vi "Chain of Responsibility Example.vi"() -> ()   [LabVIEW 2017, in "Chain of Responsiblility Example.lvlib"]
doc: "### Chain of Responsibility Example(Chain of Responsibility Example.vi)\n\n#### Overview\n\nDemonstrates the responsibility chain design pattern implemented in the CSM framework. By clicking the buttons on the front panel, you can observe how the responsibility chain processes allowed messages in a defined sequence.\n\nEach message is passed through the chain from the lowest-ordered module to the highest-ordered module. Processing stops when a module successfully handles the message, and the message is not forwarded to subsequent modules. If no module in the chain can process the message, this example returns an error.\n\n#### Introduction\n\nThis example demonstrates the responsibility chain mode in the CSM framework. Responsibility chain CSM module should always be marked with a \"$\" and an integer number as suffix, such as \"CSMName$1\", \"CSMName$2\", and so on. \n\nA group of responsibility chain CSM modules process messages both in allowed ways and also in a sequential order:\n\n- Only specially allowed messages can be processed by each individual chain module.\n- If one message is allowed by multiple chain modules, the chain module with the lowest order will process the message and the message won't be processed by higher-ordered chain module any more.\n\n#### Instructions\n\n1. Run this VI.\n2. Click any of the buttons on the front panel, such as \"Action: action 1 -> Chain\", then you can see which chain module has processed which message. \n3. Click the \"Macro: Exit -> Chain\" or \"Macro: Exit -@ Chain\" button, then you can see the chain module will be initiated in an ordered way.\n\n#### Steps\n\nStep 1: Add special allowed messages for each individual CSM submodule which will be then marked with chain mode, such as \"Action: action 1\" and \"Action: action 2\" for the \"Chain$1\" CSM submodule in this example.\n\nStep 2: Drop a template CSM VI with UI and name it as ChainModeExample. \n\nStep 3: Create boolean buttons in the UI, such as \"Action: action 1 -> Chain\" and so on to simulate the inter-module message transfer. \n\nStep 4: Use high-level APIs to monitor the status of all running CSM modules.\n\nStep 5: Use global log APIs to calculate and monitor the real-time logging capability, please refer to 4. Advance Examples\\6. Global Log Handling Capability for more details."
uses:
  Chain of Responsiblility Example.lvlib
  user.lib/_NEVSTOP/Communicable State Machine(CSM)/Utility/_support/Periodic String Filter Level.ctl
  user.lib/_NEVSTOP/Communicable State Machine(CSM)/_Support/Typedef/_CSM_MODE.ctl
  user.lib/_NEVSTOP/Communicable State Machine(CSM)/Utility/Periodic String Filter Setting.ctl
  user.lib/_NEVSTOP/Communicable State Machine(CSM)/AdvanceAPI/CSM - Revert Arguments-Safe String.vi
  user.lib/_NEVSTOP/Communicable State Machine(CSM)/AdvanceAPI/CSM - Make String Arguments Safe.vi
  user.lib/_NEVSTOP/Communicable State Machine(CSM)/AdvanceAPI/CSM - Break Down Multiple States String.vi
  user.lib/_NEVSTOP/Communicable State Machine(CSM)/AdvanceAPI/CSM - Compact Multiple States.vi
  user.lib/_NEVSTOP/Communicable State Machine(CSM)/AdvanceAPI/CSM - Keywords.vi
  user.lib/_NEVSTOP/Communicable State Machine(CSM)/_Shared/Trim Single-line Text.vi
  user.lib/_NEVSTOP/Communicable State Machine(CSM)/Communicable State Machine.lvlib
  user.lib/_NEVSTOP/Communicable State Machine(CSM)/_Shared/CSM Shared.lvlib
panel:
  out "Array":T2(array[cluster])
  in  "All?":bool
  out "LogInQ":i32
  out "State History 2":string
  out "log handling Speed(#/s)":dbl
  out "LogInQ changing Speed(#/s)":dbl
  out "Level":T3
  in  "Macro: Exit -@ Chain":bool
  in  "Macro: Exit -> Chain":bool
  in  "Action: action 6 -@ Chain":bool
  in  "Action: action 5 -@ Chain":bool
  in  "Action: action 4 -@ Chain":bool
  in  "Action: action 3 -@ Chain":bool
  in  "Action: action 2 -@ Chain":bool
  in  "Action: action 1 -@ Chain":bool
  in  "Action: action 6 -> Chain":bool
  in  "Action: action 5 -> Chain":bool
  in  "Action: action 4 -> Chain":bool
  in  "Action: action 3 -> Chain":bool
  in  "Action: action 2 -> Chain":bool
  in  "Action: action 1 -> Chain":bool
  out "State History":string
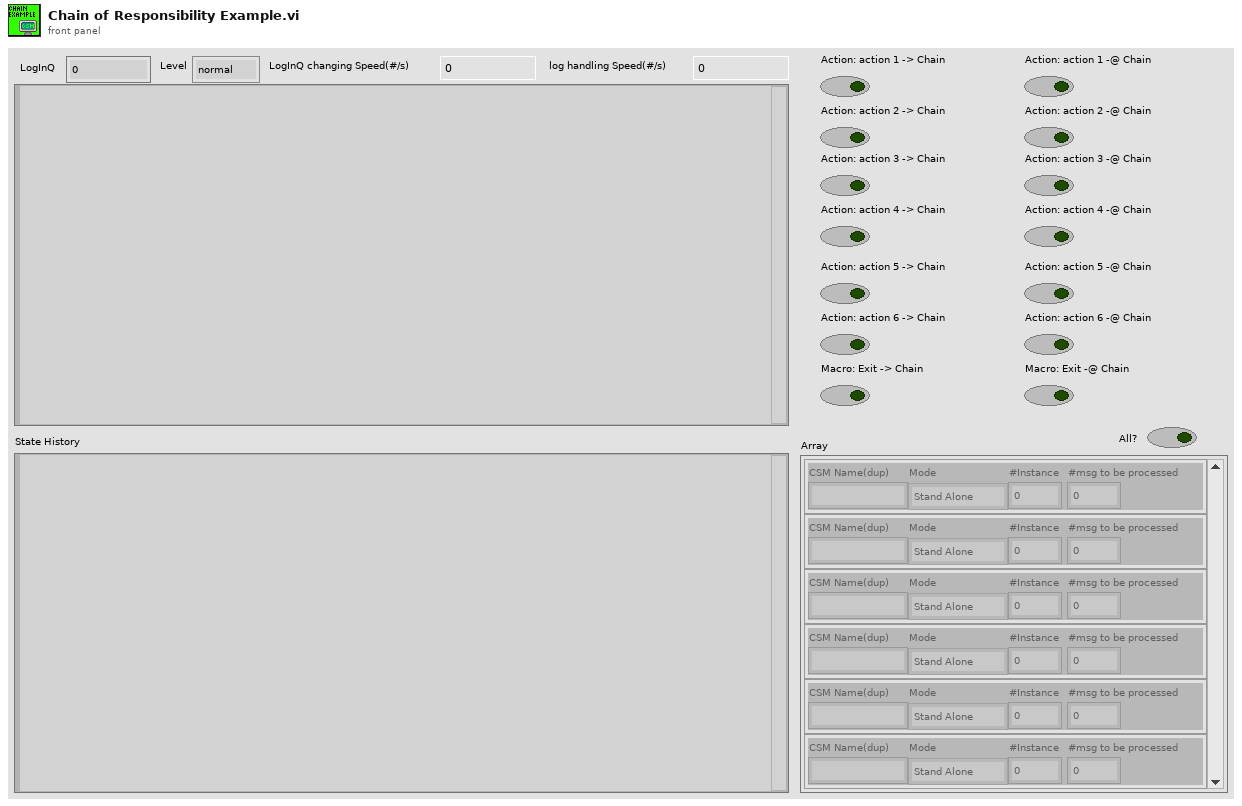
[diagram p1: front panel]
types:
  T1 = typedef "Communicable State Machine.lvlib/_CSM_MODE.ctl" = enum16{"Not Exist", "Stand Alone", "CSM", "Worker", "Worker Agent", "Chain Node", "Chain"}
  T2 = cluster{"CSM Name(dup)":string, "Mode":T1, "#Instance":i32, "#msg to be processed":i32}[]
  T3 = typedef "Communicable State Machine.lvlib/Periodic String Filter Level.ctl" = enum16{"normal", "L1", "L2", "L3", "L4"}
  T4 = enum32{"Invalid", "Standard", "Closed", "Hidden", "Minimized", "Maximized"}
  T5 = enum32{"invalid app kind", "Development System", "Run Time System", "Student Edition", "Embedded LabVIEW", "Evaluation", "Custom"}
  T6 = typedef "Communicable State Machine.lvlib/_CSM_Response Source Message.ctl" = cluster{"‘State":string, "’Arguments":string, "’Error":errorcluster}
  T7 = cluster{"Current VI Reference":refnum<vi>, "Close Panel on Exit?":bool}
  T8 = cluster{"Core":cluster{"Current VI Reference":refnum<vi>, "Close Panel on Exit?":bool}, "Your Boolean data":bool, "Your string data":string}
  T9 = cluster{"CSM Name (Dup)":string, "Mode":T1, "#Instance":i32, "#Elements In Queue":i32}
  T10 = typedef "Communicable State Machine.lvlib/Periodic String Filter Setting.ctl" = cluster{"threashold(#/s)":dbl, "Check Peroid(s)":dbl}
  T11 = typedef "Communicable State Machine.lvlib/_CSM_GlobalLog_MSG.ctl" = cluster{"Name (\"\" to Use UUID)":string, "Current State":string, "Arguments":string, "Source Message":T6, "Source Module":string, "Complete(T)/Start(F)":bool, "LogType":T12, "Time Stamp":timestamp}
  T12 = typedef "Communicable State Machine.lvlib/_CSM_GlobalLog_MSG_TYPE.ctl" = enum16{"User Log", "State Change", "Status", "Interrupt", "Register", "Unregister", "Error Log", "Module Created", "Module Destroyed"}
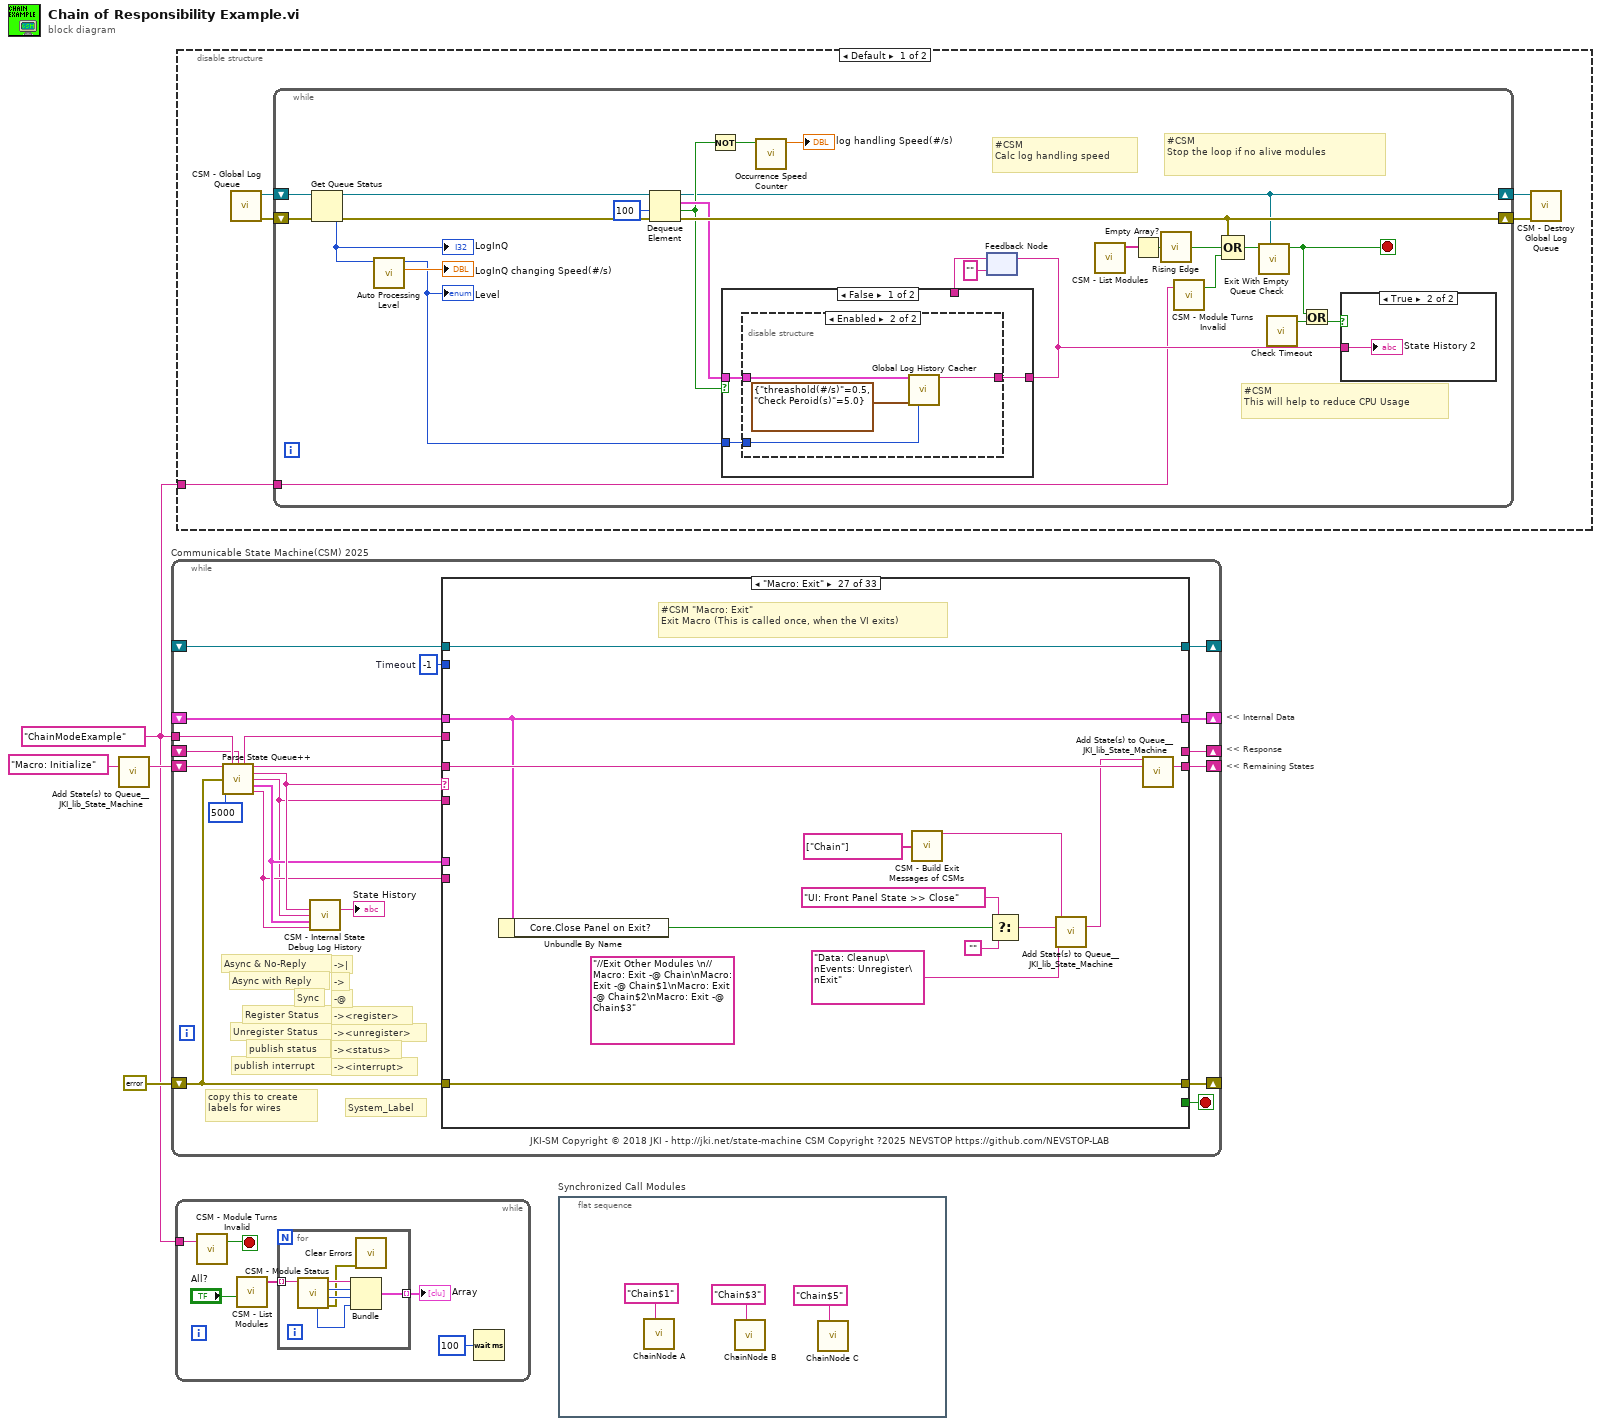
[diagram p0: block diagram]
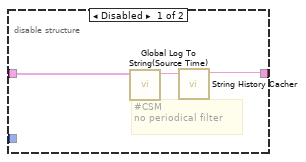
[diagram p2: hidden frame]
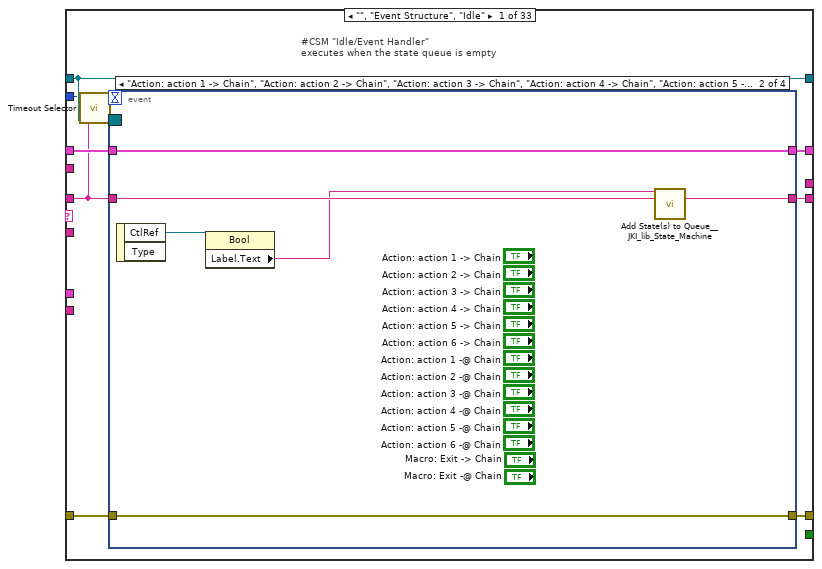
[diagram p6: hidden frame]
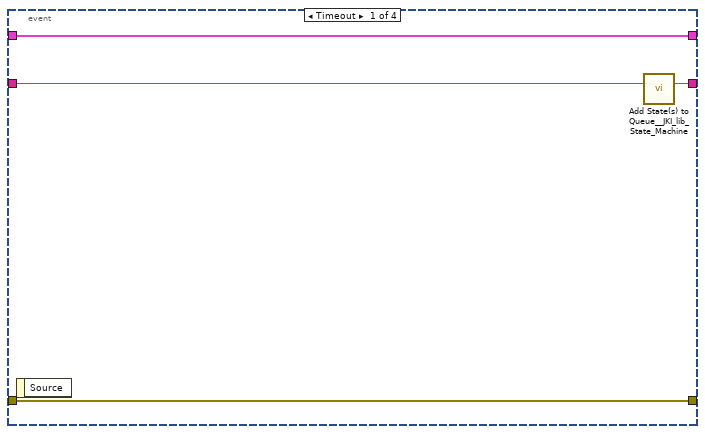
[diagram p7: hidden frame]
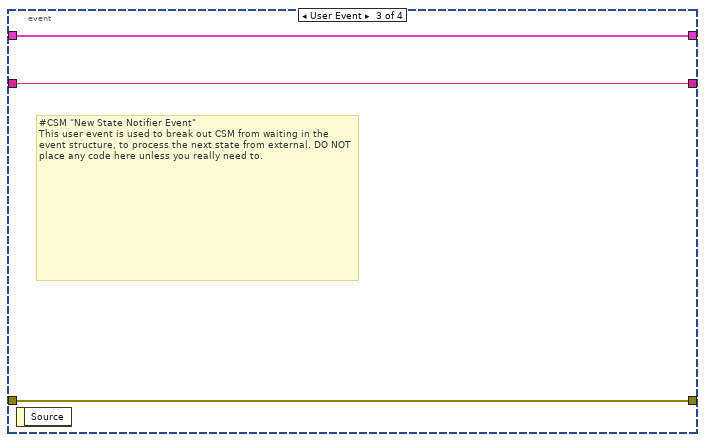
[diagram p8: hidden frame]
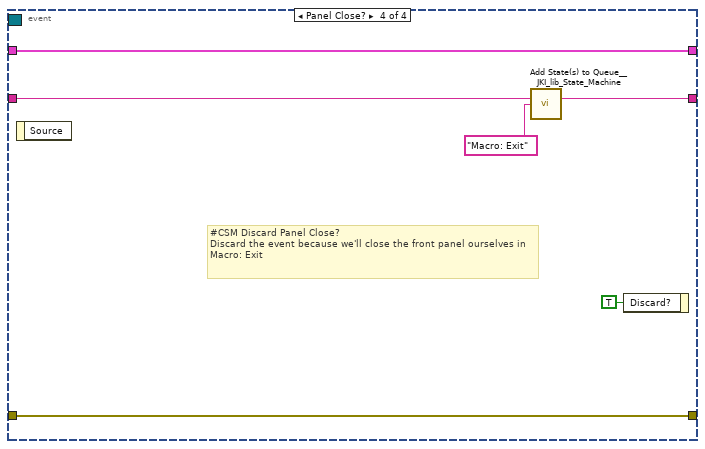
[diagram p9: hidden frame]
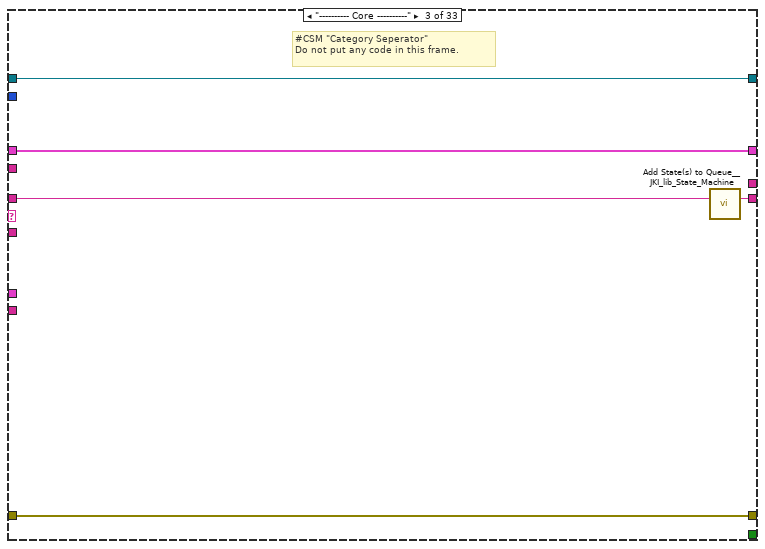
[diagram p11: hidden frame]
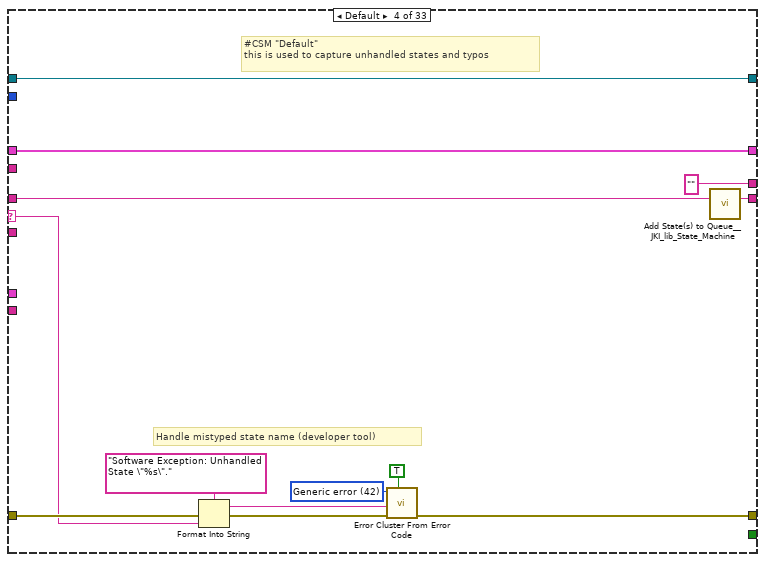
[diagram p12: hidden frame]
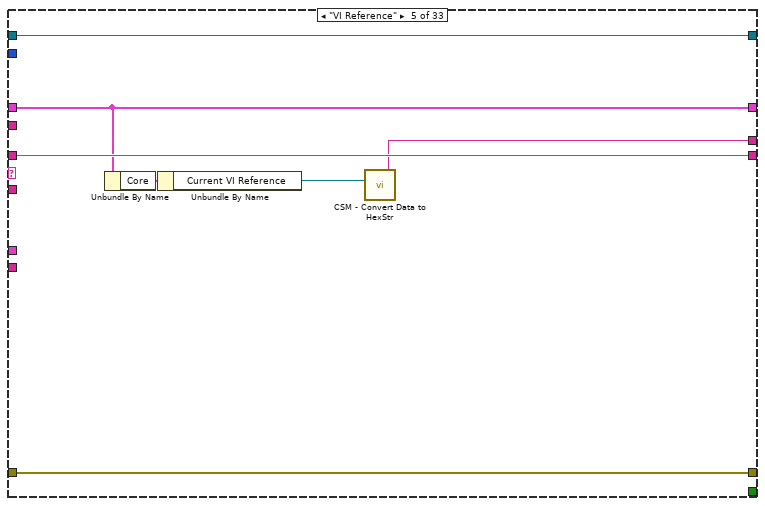
[diagram p13: hidden frame]
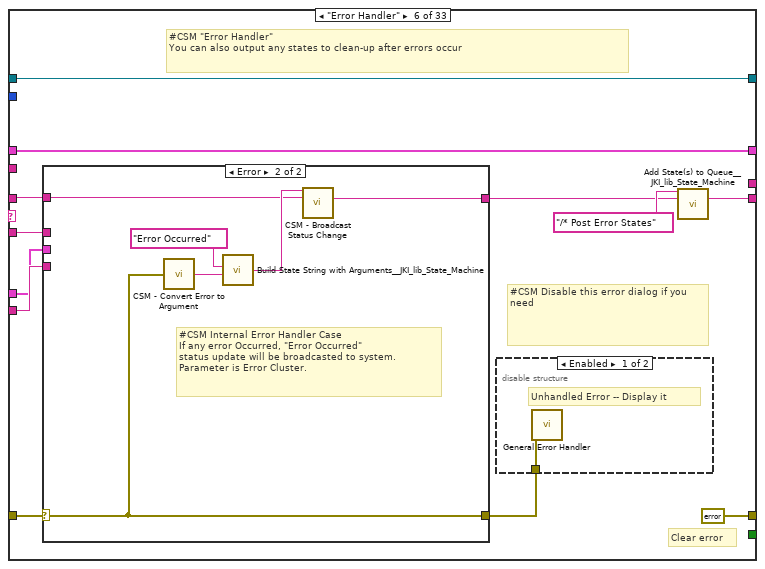
[diagram p14: hidden frame]
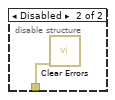
[diagram p15: hidden frame]
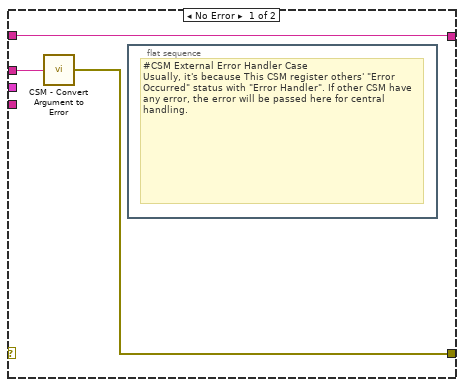
[diagram p16: hidden frame]
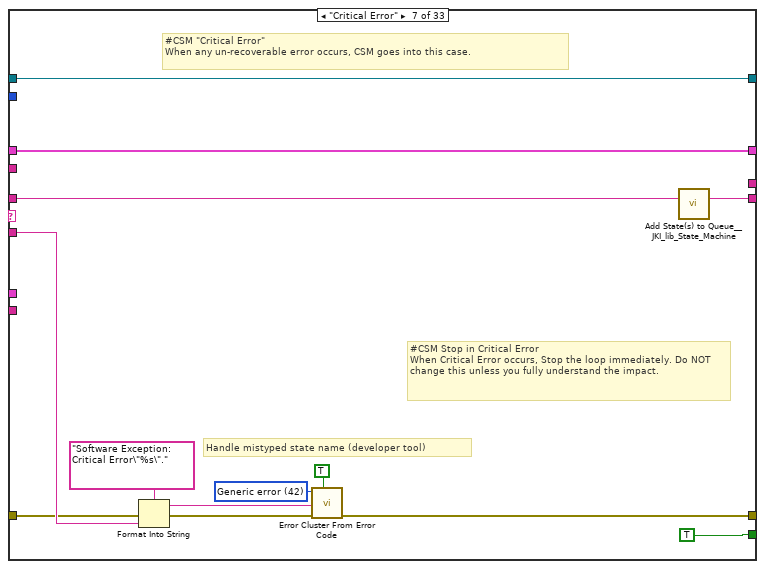
[diagram p17: hidden frame]
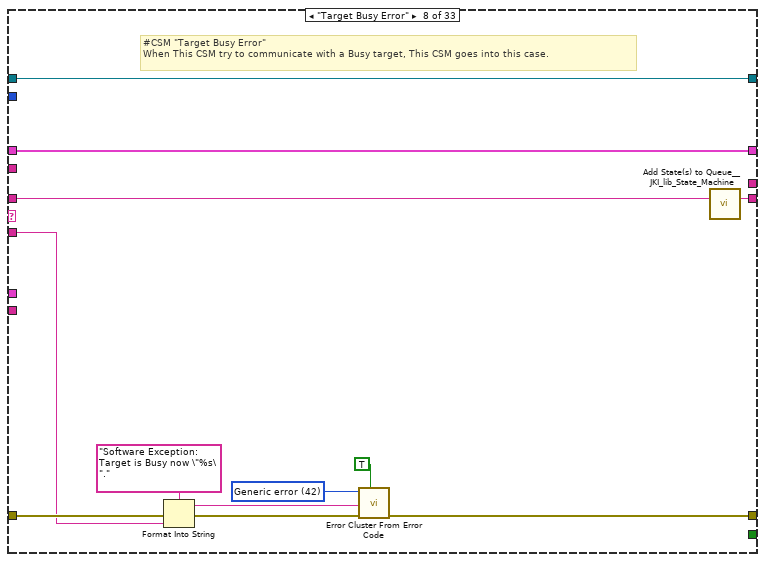
[diagram p18: hidden frame]
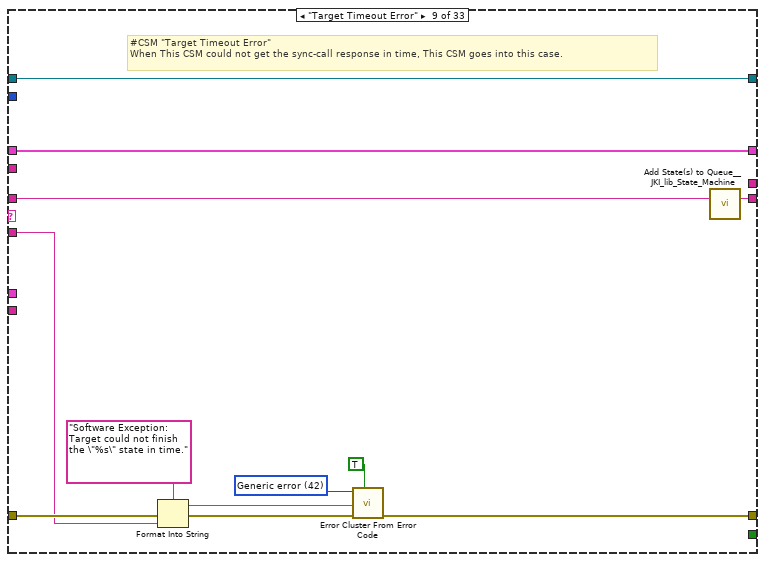
[diagram p19: hidden frame]
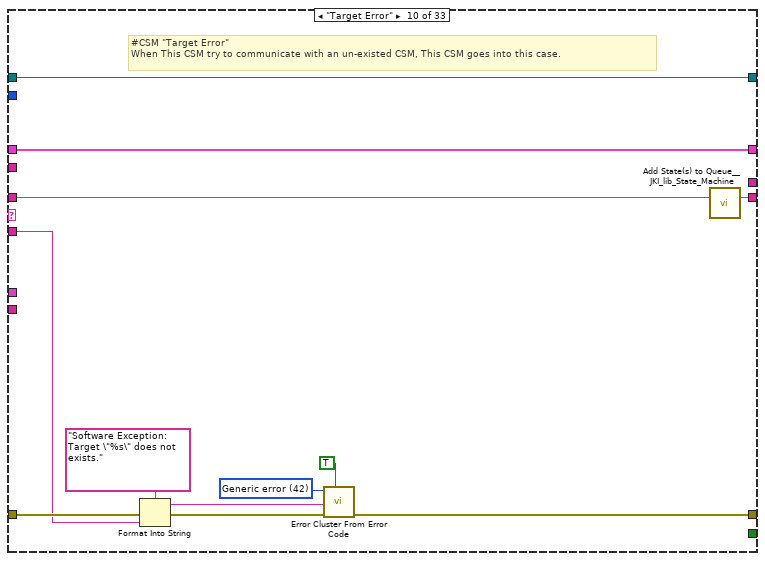
[diagram p20: hidden frame]
diagram:
  w1 = "ChainModeExample" ("Name (\"\" to Use UUID)")
  # "<< Internal Data"
  # "<< Response"
  # "<< Remaining States"
  n1 = call <vilib>:"Add State(s) to Queue__JKI_lib_State_Machine.vi"("State(s) in (\"\")"="Macro: Initialize" ("Init State(\"Macro: Initialize\")")) -> ("States Out"=w4:string)  [unwired: 14 in]
  n2 = while "Communicable State Machine(CSM) 2025" {
    shift-right: [w20] -> _
    shift-left: _ -> [w19]
    shift-right: [w23] -> _
    shift-left: errorcluster {"status"=FALSE, "code"=0, "source"=""} ("error out") -> [w17]
    shift-right: [w22] -> _
    shift-left: w4 -> [w24]
    tunnel: w1 -> [w12]
    shift-right: [w15] -> _
    shift-left: _ -> [w7]
    shift-right: [w14] -> _
    shift-left: _ -> [w13]
    stop <- w21 stop-if-true
    w18 = -1  # Timeout
    # "-><interrupt>"
    # "-><status>"
    # "-><unregister>"
    # "-><register>"
    # "-@"
    # "->"
    # "->|"
    # "publish interrupt"
    # "publish status"
    # "Unregister Status"
    # "Register Status"
    # "Sync"
    # "Async with Reply"
    # "Async & No-Reply"
    # "copy this to create labels for wires"
    # "System_Label"
    # "JKI-SM Copyright © 2018 JKI - http://jki.net/state-machine CSM Copyright ?2025 NEVSTOP https://github.com/NEVSTOP-LAB"
    n3 = call "Parse State Queue++.vi"("State Queue"=w24, "Name (\"\" to Use UUID)"=w12, "Response Arguments"=w7, "Previous Error"=w17, "Response Timeout (-2 Use Global Settings)"=5000 ("Response Timeout(1000ms)")) -> ("Name Used"=w8:string, "Remaining States"=w25:string, "Current State"=w11:string, "Arguments"=w6:string, ">> Response Source Message >>"=w10:T6, ">> Source CSM >>"=w9:string)  [unwired: 5 in]
    n4 = call "CSM - Internal State Debug Log History.vi"("State"=w11, "Arguments (\"\")"=w6, ">> Response Source Message >>"=w10, "Source (\"\")"=w9) -> ("Debug Log"=→"State History":string)  [unwired: 11 in]
    n5 = case shown="\"Macro: Exit\"" w11 {
      selector: w11 -> [_ _ _ w65 _ _ _ _ _ _ _ _ _ _ _ _ _ _ _ _ _ _ _ _ _ _ _ _ _ _ _ _ _]
      tunnel: w25 -> [w26 w57 w62 w69 w81 w87 w117 w120 w137 w149 w164 w173 w188 w194 w199 w207 w214 w219 w226 w230 w236 w241 w248 w264 w334 w340 w353 w356 w361 w365 w371 w376 w381]
      tunnel: w6 -> [_ _ _ _ _ w85 w110 w122 w133 w145 w158 _ _ _ _ _ _ _ _ _ _ _ w243 w258 _ _ _ _ _ _ _ _ _]
      tunnel: w19 -> [w33 w56 w59 w67 w80 w93 w118 w124 w135 w147 w162 w172 w181 w192 w196 _ w209 w216 w225 w229 w233 w239 w246 w260 w331 w337 w350 w355 w360 w364 w368 w373 w378]
      tunnel: [w32 w55 w60 w71 w82 errorcluster {"status"=FALSE, "code"=0, "source"=""} ("error out") w106 w119 w131 w143 w161 w174 w185 w191 w197 w204 w210 w217 w220 w228 w234 w238 w244 w261 w332 w338 w351 w357 w362 w366 w369 w374 w379] -> w23
      tunnel: w17 -> [w31 w55 w60 w70 w82 w91 w107 w126 w138 w150 _ w174 w185 w191 w197 w204 w211 w217 _ w231 w234 w238 w245 w262 w332 w338 w351 w357 w362 w366 w369 w374 w379]
      tunnel: [w34 w57 w61 w68 w81 w89 w116 w125 w136 w148 w165 w173 w187 w193 w198 w206 w213 w218 w226 w230 w235 w240 w247 w263 w333 w339 w352 w356 w361 w365 w370 w375 w380] -> w22
      tunnel: [_ _ _ _ _ _ TRUE _ _ _ _ _ _ TRUE _ _ _ _ _ _ _ _ _ _ _ _ _ _ _ _ _ _ _] -> w21
      tunnel: [w30 w56 w59 w67 w80 w93 w118 w124 w135 w147 w163 w172 w186 w192 w196 w205 w209 w216 w225 w229 w233 w239 w246 w260 w331 w337 w350 w355 w360 w364 w368 w373 w378] -> w20
      tunnel: w18 -> [w28 _ _ _ _ _ _ _ _ _ _ _ _ _ _ _ _ _ _ _ _ _ _ _ _ _ _ _ _ _ _ _ _]
      tunnel: w9 -> [_ _ _ _ _ w84 _ _ _ _ w159 _ _ _ _ _ _ _ _ _ _ _ _ _ _ _ _ _ _ _ _ _ _]
      tunnel: w10 -> [_ _ _ _ _ w83 _ _ _ _ w160 _ _ _ _ _ _ _ _ _ _ _ _ _ _ _ _ _ _ _ _ _ _]
      tunnel: [_ _ _ "" w76 _ _ _ _ _ _ _ _ _ _ _ _ _ _ _ _ _ _ _ _ _ _ _ "API1 Response" _ _ _ _] -> w15
      tunnel: [w29 w54 w58 w63 w79 w92 w108 w121 w132 w144 w166 w171 w175 w189 w195 w200 w208 w215 w224 w227 w232 w237 w242 w257 w330 w335 w343 w354 w359 w363 w367 w372 w377] -> w14
      tunnel: w13 -> [w29 w54 w58 w63 w79 w92 w108 w121 w132 w144 w166 w171 w175 w189 w195 w200 w208 w215 _ w227 w232 w237 w242 w257 w330 w335 w343 w354 w359 w363 w367 w372 w377]
      tunnel: w8 -> [_ _ _ _ _ _ _ _ _ _ _ _ _ _ _ _ _ _ w223 _ _ _ _ _ _ _ _ _ _ _ _ _ _]
      frame "", "Event Structure", "Idle" {
        # "#CSM \"Idle/Event Handler\"\nexecutes when the state queue is empty"
        n6 = call "Timeout Selector.vi"("Remaining States"=w26, "Timeout Expected"=w28) -> ("Timeout"=w27:i32)  [unwired: 5 in]
        n7 = event shown="[1] \"Action: action 1 -> Chain\", \"Action: action 2 -> Chain\", \"Action: action 3 -> Chain\", \"Action: action 4 -> Chain\", \"Action: action 5 -> Chain\", \"Action: action 6 -> Chain\", \"Action: action 1 -@ Chain\", \"Action: action 2 -@ Chain\", \"Action: action 3 -@ Chain\", \"Action: action 4 -@ Chain\", \"Action: action 5 -@ Chain\", \"Action: action 6 -@ Chain\", \"Macro: Exit -> Chain\", \"Macro: Exit -@ Chain\": Value Change" {
          selector: w29 -> [_ _ _ _]
          dyn-events: _ -> [_ _ _ _]
          timeout: w27 -> [_ _ _ _]
          tunnel: w26 -> [w38 w42 w46 w53]
          tunnel: [w37 w41 w46 w52] -> w34
          tunnel: w33 -> [w35 w43 w47 w50]
          tunnel: [w36 w44 w45 w51] -> w32
          tunnel: w31 -> [w36 w44 w45 w51]
          tunnel: [w35 w43 w47 w50] -> w30
          event Timeout {
            n8 = event-data() -> ()  [unwired: 1 in, 1 out]
            n9 = call <vilib>:"Add State(s) to Queue__JKI_lib_State_Machine.vi"("State(s) in (\"\")"=w38) -> ("States Out"=w37:string)  [unwired: 14 in]
          }
          event "Action: action 1 -> Chain", "Action: action 2 -> Chain", "Action: action 3 -> Chain", "Action: action 4 -> Chain", "Action: action 5 -> Chain", "Action: action 6 -> Chain", "Action: action 1 -@ Chain", "Action: action 2 -@ Chain", "Action: action 3 -@ Chain", "Action: action 4 -@ Chain", "Action: action 5 -@ Chain", "Action: action 6 -@ Chain", "Macro: Exit -> Chain", "Macro: Exit -@ Chain": Value Change {
            n10 = event-data() -> ("CtlRef"=w40:refnum<vi>)  [unwired: 1 in, 1 out]
            n11 = property class="Bool"(reference=w40) -> ("Label.Text"=w39:string)  [unwired: 1 in, 2 out]
            n12 = call <vilib>:"Add State(s) to Queue__JKI_lib_State_Machine.vi"("State(s) in Front (\"\")"=w39, "State(s) in (\"\")"=w42) -> ("States Out"=w41:string)  [unwired: 13 in]
          }
          event User Event {
            # "#CSM \"New State Notifier Event\"\nThis user event is used to break out CSM from waiting in the event structure, to process the next state from external. DO NOT place any code here unless you really need to."
            n13 = event-data() -> ()  [unwired: 1 in, 1 out]
          }
          event Panel Close? {
            # "#CSM Discard Panel Close?\nDiscard the event because we'll close the front panel ourselves in Macro: Exit"
            n14 = event-data() -> ()  [unwired: 1 in, 1 out]
            n15 = call <vilib>:"Add State(s) to Queue__JKI_lib_State_Machine.vi"("State(s) in (\"\")"=w53, "State(s) at Back (\"\")"="Macro: Exit") -> ("States Out"=w52:string)  [unwired: 13 in]
            n16 = event-data("Discard?"=TRUE) -> ()  [unwired: 1 in, 1 out]
          }
        }
      }
      frame "CSM Documentation" {
        # "#CSM \"Documentation\"\nCase for holding CSM Documenation"
        # "CSM Documentation"
        # "#CSM Commenting\nTo add a comment use \"//\" or \"#\" and all text to the right will be ignored\n\nCommenting Example:\nUI: Initialize // This initializes the UI\n// Another comment line"
        # "#CSM State Syntax\n\n    // Local Message Example\n    DoSth: DoA >> Arguments\n\n    // Sync Call Example\n    API: xxxx >> Arguments -@ TargetModule\n\n    // Async Call Example\n    API: xxxx >> Arguments -> TargetModule\n\n    // Async Call without Reply Example\n    API: xxxx >> Arguments ->| TargetModule\n\n    // Broadcast normal status:\n    Status >> StatusArguments  -><status>\n\n    // Broadcast Interrupt status:\n    Interrupt >> StatusArguments  -><interrupt>\n\n    // Register Source Module's status to Handler Module\n    Status@Source Module >> Handler Module@Handler Module -><register>\n\n    // Unegister Source Module's status\n    Status@Source Module >> Handler Module -><unregister>"
        # "#CSM README FIRST\n\nCSM is a LabVIEW application framework that builds upon JKI State Machine (CSM). It follows the pattern of CSM and extends the keywords to describe message communication between CSM modules, including concepts such as Sync-Message, Async-Message, Subscription/Unsubscription of status - essential elements for creating reusable code modules. For more information, please visit the CSM wiki: https://github.com/NEVSTOP-LAB/JKI-State-Machine-Plus-Plus/wiki\n\nFor instructions on JKI State Machine, visit: \n    http://jki.net/state-machine/\nFor information about CSM, visit: \n    https://github.com/NEVSTOP-LAB"
      }
      frame "---------- Core ----------" {
        # "#CSM \"Category Seperator\"\nDo not put any code in this frame."
        n17 = call <vilib>:"Add State(s) to Queue__JKI_lib_State_Machine.vi"("State(s) in (\"\")"=w62) -> ("States Out"=w61:string)  [unwired: 14 in]
      }
      frame Default {
        w74 = 42 items=["No error", "Argument error", "Memory is full", "Out of zone", "End of file", "File already open", "Generic file I/O error", "File not found", "File permission error", "Disk is full", "Duplicate path", "Too many files open", "System feature not enabled", "Resource file not found", "Cannot add resource", "Resource not found", "Image not found", "Image memory error", "Pen does not exist", "Config type invalid", "Config token not found", "Config parse error", "Config memory error", "Bad external code format", "Bad external code offset", "External code not present", "Null window", "Destroy window error", "Null menu", "Print aborted", "Bad print record", "Print driver error", "Windows error during printing", "Memory error during printing", "Print dialog error", "Generic print error", "Invalid device refnum", "Device not found", "Device parameter error", "Device unit error", "Cannot open device", "Device call aborted", "Generic error", "Cancelled by user", "Object ID too low", "Object ID too high", "Object not in heap", "Unknown heap", "Unknown object (invalid DefProc)", "Unknown object (DefProc not in table)", "Message out of range", "Invalid (null) method", "Unknown message", "Manager call not supported", "Bad address", "Network operation in progress", "Network operation timed out", "Connection is busy", "Network attribute not supported", "Network error", "Address in use", "System out of memory", "Connection aborted", "Connection refused", "Not connected", "Already connected", "Connection closed", "Initialization error (interapplication manager)", "Bad occurrence", "Wait on unbound occurrence handler", "Occurrence queue overflow", "Datalog type conflict", "Unused", "Unrecognized type (interapplication manager)", "Memory corrupt", "Failed to make temporary DLL", "Old CIN version", "Drag socket not found", "Failed to load drop-object", "Failed to register OLE object", "Failed to release OLE object", "Format specifier type mismatch", "Unknown format specifier", "Too few format specifiers", "Too many format specifiers", "Scan failed", "Newer CIN version", "Error converting to variant", "Runtime menu error", "Password tampered", "Variant attribute not found", "Incompatible variant data type", "Event data is not available", "Event Store is not present", "Occurrence is not found", "Event Queue is not created", "Event info is not available", "Refnum passed is NULL", "Error retrieving Class GUID", "Error retrieving CoClass GUID", "Error retrieving TypeLib GUID.", "Bad built application magic bytes.", "Specific driver is different from the specific driver associated with the Logical Name.", "There is no session opened to the class driver.", "Max Error", "MAX - Error with config objects", "MAX - Error loading configuration", "MAX - Group not supported"]
        # "#CSM \"Default\"\nthis is used to capture unhandled states and typos"
        # "Handle mistyped state name (developer tool)"
        n18 = Format Into String(format string="Software Exception: Unhandled State \"%s\"." ("message"), error in=w70, w65) -> (resulting string=w73:string, error out=w72:errorcluster)  [unwired: 1 in]
        n19 = call <vilib>:"Error Cluster From Error Code.vi"("show call chain? (False)"=TRUE, "error in (no error)"=w72, "error message (\"\")"=w73, "error code (0)"=w74) -> ("error out"=w71:errorcluster)  [unwired: 5 in]
        n20 = call <vilib>:"Add State(s) to Queue__JKI_lib_State_Machine.vi"("State(s) in (\"\")"=w69) -> ("States Out"=w68:string)  [unwired: 14 in]
      }
      frame "VI Reference" {
        n21 = Unbundle By Name(w80) -> ("Core"=w78:T7)
        n22 = Unbundle By Name(w78) -> ("Current VI Reference"=w77:refnum<vi>)
        n23 = call "CSM - Convert Data to HexStr.vi"("Variant"=w77) -> ("HEX String (0-9,A-F)"=w76:string)  [unwired: 8 in]
      }
      frame "Error Handler" {
        # "#CSM Disable this error dialog if you need"
        # "#CSM \"Error Handler\"\nYou can also output any states to clean-up after errors occur"
        # "Clear error"
        n24 = case shown="Error" w91 {
          selector: w91 -> [_ w100]
          tunnel: [w98 w102] -> w88
          tunnel: w87 -> [w98 w101]
          tunnel: [w97 w100] -> w86
          tunnel: w85 -> [w99 _]
          tunnel: w84 -> [_ _]
          tunnel: w83 -> [_ _]
          frame No Error {
            n25 = call "CSM - Convert Argument to Error.vi"("Argument"=w99) -> ("Error"=w97:errorcluster)  [unwired: 4 in]
            n26 = flat-sequence {
              frame #0 {
                # "#CSM External Error Handler Case\nUsually, it's because This CSM register others' \"Error Occurred\" status with \"Error Handler\". If other CSM have any error, the error will be passed here for central handling."
              }
            }
          }
          frame Error {
            # "#CSM Internal Error Handler Case \nIf any error Occurred, \"Error Occurred\" \nstatus update will be broadcasted to system.\nParameter is Error Cluster."
            n27 = call "CSM - Convert Error to Argument.vi"("Error"=w100) -> ("Argument"=w104:string)  [unwired: 4 in]
            n28 = call <vilib>:"Build State String with Arguments__JKI_lib_State_Machine.vi"("Arguments (\"\")"=w104, "State"="Error Occurred" ("Status with Arguments")) -> ("State with Arguments"=w103:string)  [unwired: 4 in]
            n29 = call "CSM - Broadcast Status Change.vi"("Status With Arguments"=w103, "State Queue"=w101) -> ("Remaining States"=w102:string)  [unwired: 13 in]
          }
        }
        n30 = disable-structure shown="Enabled" {
          disable-tunnel: w86 -> [w95 w96]
          frame Enabled {
            # "Unhandled Error -- Display it"
            n31 = call <vilib>:"General Error Handler.vi"("error in (no error)"=w95) -> ()  [unwired: 10 in, 5 out]
          }
          frame Disabled {
            n32 = call <vilib>:"Clear Errors.vi"("error in (no error)"=w96) -> ()  [unwired: 5 in, 2 out]
          }
        }
        n33 = call <vilib>:"Add State(s) to Queue__JKI_lib_State_Machine.vi"("State(s) in Front (\"\")"="/* Post Error States", "State(s) in (\"\")"=w88) -> ("States Out"=w89:string)  [unwired: 13 in]
      }
      frame "Critical Error" {
        w114 = 42 items=["No error", "Argument error", "Memory is full", "Out of zone", "End of file", "File already open", "Generic file I/O error", "File not found", "File permission error", "Disk is full", "Duplicate path", "Too many files open", "System feature not enabled", "Resource file not found", "Cannot add resource", "Resource not found", "Image not found", "Image memory error", "Pen does not exist", "Config type invalid", "Config token not found", "Config parse error", "Config memory error", "Bad external code format", "Bad external code offset", "External code not present", "Null window", "Destroy window error", "Null menu", "Print aborted", "Bad print record", "Print driver error", "Windows error during printing", "Memory error during printing", "Print dialog error", "Generic print error", "Invalid device refnum", "Device not found", "Device parameter error", "Device unit error", "Cannot open device", "Device call aborted", "Generic error", "Cancelled by user", "Object ID too low", "Object ID too high", "Object not in heap", "Unknown heap", "Unknown object (invalid DefProc)", "Unknown object (DefProc not in table)", "Message out of range", "Invalid (null) method", "Unknown message", "Manager call not supported", "Bad address", "Network operation in progress", "Network operation timed out", "Connection is busy", "Network attribute not supported", "Network error", "Address in use", "System out of memory", "Connection aborted", "Connection refused", "Not connected", "Already connected", "Connection closed", "Initialization error (interapplication manager)", "Bad occurrence", "Wait on unbound occurrence handler", "Occurrence queue overflow", "Datalog type conflict", "Unused", "Unrecognized type (interapplication manager)", "Memory corrupt", "Failed to make temporary DLL", "Old CIN version", "Drag socket not found", "Failed to load drop-object", "Failed to register OLE object", "Failed to release OLE object", "Format specifier type mismatch", "Unknown format specifier", "Too few format specifiers", "Too many format specifiers", "Scan failed", "Newer CIN version", "Error converting to variant", "Runtime menu error", "Password tampered", "Variant attribute not found", "Incompatible variant data type", "Event data is not available", "Event Store is not present", "Occurrence is not found", "Event Queue is not created", "Event info is not available", "Refnum passed is NULL", "Error retrieving Class GUID", "Error retrieving CoClass GUID", "Error retrieving TypeLib GUID.", "Bad built application magic bytes.", "Specific driver is different from the specific driver associated with the Logical Name.", "There is no session opened to the class driver.", "Max Error", "MAX - Error with config objects", "MAX - Error loading configuration", "MAX - Group not supported"]
        # "#CSM \"Critical Error\"\nWhen any un-recoverable error occurs, CSM goes into this case."
        # "#CSM Stop in Critical Error\nWhen Critical Error occurs, Stop the loop immediately. Do NOT change this unless you fully understand the impact."
        # "Handle mistyped state name (developer tool)"
        n34 = Format Into String(format string="Software Exception: Critical Error\"%s\"." ("message"), error in=w107, w110) -> (resulting string=w113:string, error out=w112:errorcluster)  [unwired: 1 in]
        n35 = call <vilib>:"Error Cluster From Error Code.vi"("show call chain? (False)"=TRUE, "error in (no error)"=w112, "error message (\"\")"=w113, "error code (0)"=w114) -> ("error out"=w106:errorcluster)  [unwired: 5 in]
        n36 = call <vilib>:"Add State(s) to Queue__JKI_lib_State_Machine.vi"("State(s) in (\"\")"=w117) -> ("States Out"=w116:string)  [unwired: 14 in]
      }
      frame "Target Busy Error" {
        w129 = 42 items=["No error", "Argument error", "Memory is full", "Out of zone", "End of file", "File already open", "Generic file I/O error", "File not found", "File permission error", "Disk is full", "Duplicate path", "Too many files open", "System feature not enabled", "Resource file not found", "Cannot add resource", "Resource not found", "Image not found", "Image memory error", "Pen does not exist", "Config type invalid", "Config token not found", "Config parse error", "Config memory error", "Bad external code format", "Bad external code offset", "External code not present", "Null window", "Destroy window error", "Null menu", "Print aborted", "Bad print record", "Print driver error", "Windows error during printing", "Memory error during printing", "Print dialog error", "Generic print error", "Invalid device refnum", "Device not found", "Device parameter error", "Device unit error", "Cannot open device", "Device call aborted", "Generic error", "Cancelled by user", "Object ID too low", "Object ID too high", "Object not in heap", "Unknown heap", "Unknown object (invalid DefProc)", "Unknown object (DefProc not in table)", "Message out of range", "Invalid (null) method", "Unknown message", "Manager call not supported", "Bad address", "Network operation in progress", "Network operation timed out", "Connection is busy", "Network attribute not supported", "Network error", "Address in use", "System out of memory", "Connection aborted", "Connection refused", "Not connected", "Already connected", "Connection closed", "Initialization error (interapplication manager)", "Bad occurrence", "Wait on unbound occurrence handler", "Occurrence queue overflow", "Datalog type conflict", "Unused", "Unrecognized type (interapplication manager)", "Memory corrupt", "Failed to make temporary DLL", "Old CIN version", "Drag socket not found", "Failed to load drop-object", "Failed to register OLE object", "Failed to release OLE object", "Format specifier type mismatch", "Unknown format specifier", "Too few format specifiers", "Too many format specifiers", "Scan failed", "Newer CIN version", "Error converting to variant", "Runtime menu error", "Password tampered", "Variant attribute not found", "Incompatible variant data type", "Event data is not available", "Event Store is not present", "Occurrence is not found", "Event Queue is not created", "Event info is not available", "Refnum passed is NULL", "Error retrieving Class GUID", "Error retrieving CoClass GUID", "Error retrieving TypeLib GUID.", "Bad built application magic bytes.", "Specific driver is different from the specific driver associated with the Logical Name.", "There is no session opened to the class driver.", "Max Error", "MAX - Error with config objects", "MAX - Error loading configuration", "MAX - Group not supported"]
        # "#CSM \"Target Busy Error\"\nWhen This CSM try to communicate with a Busy target, This CSM goes into this case."
        n37 = Format Into String(format string="Software Exception: Target is Busy now \"%s\"." ("message"), error in=w126, w122) -> (resulting string=w128:string, error out=w127:errorcluster)  [unwired: 1 in]
        n38 = call <vilib>:"Error Cluster From Error Code.vi"("show call chain? (False)"=TRUE, "error in (no error)"=w127, "error message (\"\")"=w128, "error code (0)"=w129) -> ("error out"=w119:errorcluster)  [unwired: 5 in]
        n39 = call <vilib>:"Add State(s) to Queue__JKI_lib_State_Machine.vi"("State(s) in (\"\")"=w120) -> ("States Out"=w125:string)  [unwired: 14 in]
      }
      frame "Target Timeout Error" {
        w141 = 42 items=["No error", "Argument error", "Memory is full", "Out of zone", "End of file", "File already open", "Generic file I/O error", "File not found", "File permission error", "Disk is full", "Duplicate path", "Too many files open", "System feature not enabled", "Resource file not found", "Cannot add resource", "Resource not found", "Image not found", "Image memory error", "Pen does not exist", "Config type invalid", "Config token not found", "Config parse error", "Config memory error", "Bad external code format", "Bad external code offset", "External code not present", "Null window", "Destroy window error", "Null menu", "Print aborted", "Bad print record", "Print driver error", "Windows error during printing", "Memory error during printing", "Print dialog error", "Generic print error", "Invalid device refnum", "Device not found", "Device parameter error", "Device unit error", "Cannot open device", "Device call aborted", "Generic error", "Cancelled by user", "Object ID too low", "Object ID too high", "Object not in heap", "Unknown heap", "Unknown object (invalid DefProc)", "Unknown object (DefProc not in table)", "Message out of range", "Invalid (null) method", "Unknown message", "Manager call not supported", "Bad address", "Network operation in progress", "Network operation timed out", "Connection is busy", "Network attribute not supported", "Network error", "Address in use", "System out of memory", "Connection aborted", "Connection refused", "Not connected", "Already connected", "Connection closed", "Initialization error (interapplication manager)", "Bad occurrence", "Wait on unbound occurrence handler", "Occurrence queue overflow", "Datalog type conflict", "Unused", "Unrecognized type (interapplication manager)", "Memory corrupt", "Failed to make temporary DLL", "Old CIN version", "Drag socket not found", "Failed to load drop-object", "Failed to register OLE object", "Failed to release OLE object", "Format specifier type mismatch", "Unknown format specifier", "Too few format specifiers", "Too many format specifiers", "Scan failed", "Newer CIN version", "Error converting to variant", "Runtime menu error", "Password tampered", "Variant attribute not found", "Incompatible variant data type", "Event data is not available", "Event Store is not present", "Occurrence is not found", "Event Queue is not created", "Event info is not available", "Refnum passed is NULL", "Error retrieving Class GUID", "Error retrieving CoClass GUID", "Error retrieving TypeLib GUID.", "Bad built application magic bytes.", "Specific driver is different from the specific driver associated with the Logical Name.", "There is no session opened to the class driver.", "Max Error", "MAX - Error with config objects", "MAX - Error loading configuration", "MAX - Group not supported"]
        # "#CSM \"Target Timeout Error\"\nWhen This CSM could not get the sync-call response in time, This CSM goes into this case."
        n40 = Format Into String(format string="Software Exception: Target could not finish the \"%s\" state in time." ("message"), error in=w138, w133) -> (resulting string=w140:string, error out=w139:errorcluster)  [unwired: 1 in]
        n41 = call <vilib>:"Error Cluster From Error Code.vi"("show call chain? (False)"=TRUE, "error in (no error)"=w139, "error message (\"\")"=w140, "error code (0)"=w141) -> ("error out"=w131:errorcluster)  [unwired: 5 in]
        n42 = call <vilib>:"Add State(s) to Queue__JKI_lib_State_Machine.vi"("State(s) in (\"\")"=w137) -> ("States Out"=w136:string)  [unwired: 14 in]
      }
      frame "Target Error" {
        w153 = 42 items=["No error", "Argument error", "Memory is full", "Out of zone", "End of file", "File already open", "Generic file I/O error", "File not found", "File permission error", "Disk is full", "Duplicate path", "Too many files open", "System feature not enabled", "Resource file not found", "Cannot add resource", "Resource not found", "Image not found", "Image memory error", "Pen does not exist", "Config type invalid", "Config token not found", "Config parse error", "Config memory error", "Bad external code format", "Bad external code offset", "External code not present", "Null window", "Destroy window error", "Null menu", "Print aborted", "Bad print record", "Print driver error", "Windows error during printing", "Memory error during printing", "Print dialog error", "Generic print error", "Invalid device refnum", "Device not found", "Device parameter error", "Device unit error", "Cannot open device", "Device call aborted", "Generic error", "Cancelled by user", "Object ID too low", "Object ID too high", "Object not in heap", "Unknown heap", "Unknown object (invalid DefProc)", "Unknown object (DefProc not in table)", "Message out of range", "Invalid (null) method", "Unknown message", "Manager call not supported", "Bad address", "Network operation in progress", "Network operation timed out", "Connection is busy", "Network attribute not supported", "Network error", "Address in use", "System out of memory", "Connection aborted", "Connection refused", "Not connected", "Already connected", "Connection closed", "Initialization error (interapplication manager)", "Bad occurrence", "Wait on unbound occurrence handler", "Occurrence queue overflow", "Datalog type conflict", "Unused", "Unrecognized type (interapplication manager)", "Memory corrupt", "Failed to make temporary DLL", "Old CIN version", "Drag socket not found", "Failed to load drop-object", "Failed to register OLE object", "Failed to release OLE object", "Format specifier type mismatch", "Unknown format specifier", "Too few format specifiers", "Too many format specifiers", "Scan failed", "Newer CIN version", "Error converting to variant", "Runtime menu error", "Password tampered", "Variant attribute not found", "Incompatible variant data type", "Event data is not available", "Event Store is not present", "Occurrence is not found", "Event Queue is not created", "Event info is not available", "Refnum passed is NULL", "Error retrieving Class GUID", "Error retrieving CoClass GUID", "Error retrieving TypeLib GUID.", "Bad built application magic bytes.", "Specific driver is different from the specific driver associated with the Logical Name.", "There is no session opened to the class driver.", "Max Error", "MAX - Error with config objects", "MAX - Error loading configuration", "MAX - Group not supported"]
        # "#CSM \"Target Error\"\nWhen This CSM try to communicate with an un-existed CSM, This CSM goes into this case."
        n43 = Format Into String(format string="Software Exception: Target \"%s\" does not exists." ("message"), error in=w150, w145) -> (resulting string=w152:string, error out=w151:errorcluster)  [unwired: 1 in]
        n44 = call <vilib>:"Error Cluster From Error Code.vi"("show call chain? (False)"=TRUE, "error in (no error)"=w151, "error message (\"\")"=w152, "error code (0)"=w153) -> ("error out"=w143:errorcluster)  [unwired: 5 in]
        n45 = call <vilib>:"Add State(s) to Queue__JKI_lib_State_Machine.vi"("State(s) in (\"\")"=w149) -> ("States Out"=w148:string)  [unwired: 14 in]
      }
      frame "Async Response", "Response" {
        # "#CSM \"Async Response\"\nHandle Async-call Response (\"Async Response\" for ->)"
        # "#CSM \"Response\"\nHandle Sync-call Response (\"Response\" for -@)"
        n46 = Unbundle(w160) -> ("‘State"=w157:string, "’Arguments"=w156:string, "’Error"=w155:errorcluster)
        n47 = case shown="Default" w157 {
          tunnel: [w167] -> w165
          tunnel: w164 -> [w168]
          tunnel: [w170] -> w163
          tunnel: w162 -> [w170]
          tunnel: [w169] -> w161
          tunnel: w155 -> [w169]
          tunnel: w159 -> [_]
          tunnel: w158 -> [_]
          tunnel: w156 -> [_]
          frame Default {
            # "#CSM Response Comments\nAfter Message is executed, CSM goes to this state for receive the response.\n    For Async Message(->), \"Async Response\" is used. This CSM will goes to \"Async Message Posted\" immediately and receive the \"Async Response\" after the callee finishes the message.\n    For Sync Message(@),  This CSM will wait until the message is done and immediately goes to \"Response\""
            n48 = call <vilib>:"Add State(s) to Queue__JKI_lib_State_Machine.vi"("State(s) in (\"\")"=w168) -> ("States Out"=w167:string)  [unwired: 14 in]
          }
        }
      }
      frame "Async Message Posted" {
        # "#CSM \"Async Message Posted\"\nAfter Async Message is posted (-> or ->| ), CSM goes to this state for post-action.\nYou can use Argument - State to tell which Async Message is called."
      }
      frame "Initialize Core Data" {
        # "#CSM \"Initialize Core Data\"\nThis is used to determine panel behavior on exit"
        # "originally closed?"
        # "exe?"
        # "If panel starts closed or is an EXE, then close it when we exit"
        n49 = property class="VI"() -> ("FP.State"=w178:T4)  [unwired: 2 in, 2 out]
        n50 = property class="App"() -> ("App.Kind"=w184:T5)  [unwired: 2 in, 2 out]
        n51 = control-ref of="Current VI Reference"() -> (w179:refnum<vi>)
        n52 = Equal?(x=w178, y=T4."Closed" ("Front Panel Window:State")) -> (x = y?=w176:bool)
        n53 = Equal?(x=w184, y=T5."Run Time System" ("Application:Kind")) -> (x = y?=w182:bool)
        n54 = Or(x=w176, y=w182) -> (x .or. y?=w180:bool)
        n55 = Bundle By Name(cluster=w181, "Core.Current VI Reference"=w179, "Core.Close Panel on Exit?"=w180) -> (w186:T8)
        n56 = call <vilib>:"Add State(s) to Queue__JKI_lib_State_Machine.vi"("State(s) in (\"\")"=w188) -> ("States Out"=w187:string)  [unwired: 14 in]
      }
      frame "Exit" {
        # "#CSM \"Exit\"\nCase for exiting the loop. No errors that occur here will be handled."
        n57 = call <vilib>:"Add State(s) to Queue__JKI_lib_State_Machine.vi"("State(s) in (\"\")"=w194) -> ("States Out"=w193:string)  [unwired: 14 in]
      }
      frame "---------- Data ----------" {
        # "#CSM \"Category Seperator\"\nDo not put any code in this frame."
        n58 = call <vilib>:"Add State(s) to Queue__JKI_lib_State_Machine.vi"("State(s) in (\"\")"=w199) -> ("States Out"=w198:string)  [unwired: 14 in]
      }
      frame "Data: Initialize" {
        w201 = T7 {"Current VI Reference"=refnum, "Close Panel on Exit?"=FALSE}  # Core
        w203 = TRUE  # Your Boolean data
        w202 = ""  # Your string data
        # "do not delete - used by framework"
        # "Expand Bundle to add new data elements to shift register data."
        # "Add new data here."
        # "Data names and types of shift register data are defined by this bundle."
        # "#CSM \"Data: Initialize\"\nInitialize the shift-register data, here.\n(data names are defined by what you wire into the bundle function)"
        n59 = Bundle("Core"=w201, "Your Boolean data"=w203, "Your string data"=w202) -> (w205:T8)  [unwired: 1 in]
        n60 = call <vilib>:"Add State(s) to Queue__JKI_lib_State_Machine.vi"("State(s) in (\"\")"=w207) -> ("States Out"=w206:string)  [unwired: 14 in]
      }
      frame "Data: Cleanup" {
        # "#CSM \"Data: Cleanup\"\nCleanup any data and references, here.\n(this is called automatically, by the Macro: Exit)"
        n61 = Unbundle By Name(w209) -> ("Core.Current VI Reference"=w212:refnum<vi>)
        n62 = Close Reference(reference=w212, error in (no error)=w211) -> (error out=w210:errorcluster)
        n63 = call <vilib>:"Add State(s) to Queue__JKI_lib_State_Machine.vi"("State(s) in (\"\")"=w214) -> ("States Out"=w213:string)  [unwired: 14 in]
      }
      frame "---------- Events ----------" {
        # "#CSM \"Category Seperator\"\nDo not put any code in this frame."
        n64 = call <vilib>:"Add State(s) to Queue__JKI_lib_State_Machine.vi"("State(s) in (\"\")"=w219) -> ("States Out"=w218:string)  [unwired: 14 in]
      }
      frame "Events: Register" {
        # "#CSM \"Events: Register\"\nRegister user event. New Message Event is registered to break CSM waiting in event structure by default."
        # "#CSM Register New Message Event\nRegister message event to break Waiting in Event structure."
        n65 = call "CSM - Get New State Notifier Event.vi"("Name (\"\" to Use UUID) In"=w223) -> ("error out"=w221:errorcluster, "New State Notifier Event"=w222:refnum<user-event>)  [unwired: 9 in]
        n66 = register-events(error in=w221, w222) -> (reference out=w224:refnum<event-registration>, error out=w220:errorcluster)  [unwired: 1 in]
      }
      frame "Events: Unregister" {
        # "#CSM \"Events: Unregister\"\nUnregister user event."
        n67 = Unregister For Events(event registration refnum=w227, error in=w231) -> (error out=w228:errorcluster)
      }
      frame "---------- UI ----------" {
        # "#CSM \"Category Seperator\"\nDo not put any code in this frame."
        n68 = call <vilib>:"Add State(s) to Queue__JKI_lib_State_Machine.vi"("State(s) in (\"\")"=w236) -> ("States Out"=w235:string)  [unwired: 14 in]
      }
      frame "UI: Initialize" {
        # "#CSM \"UI: Initialize\"\nInitialize the User Interface, here.\n(this is called automatically, by the Macro: Init)"
        n69 = call <vilib>:"Add State(s) to Queue__JKI_lib_State_Machine.vi"("State(s) in (\"\")"=w241) -> ("States Out"=w240:string)  [unwired: 14 in]
      }
      frame "UI: Cursor Set" {
        # "Argument"
        # "#CSM \"UI: Cursor Set\"\nSet and Unset Cursor Busy.\n(Usage: \"UI: Cursor Set >> Busy|Idle\")"
        n70 = disable-structure shown="Default" {
          disable-tunnel: w245 -> [w251 w256]
          disable-tunnel: [w250 w256] -> w244
          disable-tunnel: w243 -> [w249 _]
          frame condition #0 (active) {
            n71 = case shown="\"Busy\"" w249 {
              tunnel: w251 -> [w253 w255]
              tunnel: [w252 w254] -> w250
              frame "Idle", Default {
                n72 = call <vilib>:"Unset Busy.vi"("error in (no error)"=w253) -> ("error out"=w252:errorcluster)  [unwired: 10 in]
              }
              frame "Busy" {
                n73 = call <vilib>:"Set Busy.vi"("error in (no error)"=w255) -> ("error out"=w254:errorcluster)  [unwired: 9 in, 1 out]
              }
            }
          }
          frame condition #1 {
          }
        }
        n74 = call <vilib>:"Add State(s) to Queue__JKI_lib_State_Machine.vi"("State(s) in (\"\")"=w248) -> ("States Out"=w247:string)  [unwired: 14 in]
      }
      frame "UI: Front Panel State" {
        # "Argument"
        # "#CSM \"UI: Front Panel State\"\nSet Front Panel Open or Closed\n(Usage: \"UI: Front Panel State >> Open|Close\")"
        n75 = Unbundle By Name(w260) -> ("Core.Current VI Reference"=w259:refnum<vi>)
        n76 = case shown="\"Minimize\", \"Minimized\"" w258 {
          tunnel: w262 -> [w270 w285 w296 w309 w322]
          tunnel: [w272 w286 w298 w311 w324] -> w261
          tunnel: w259 -> [w271 w283 w297 w310 w323]
          frame "Open", "Standard", Default {
            w265 = T4."Standard" ("State")
            n77 = property class="VI"(reference=w271, error in=w270) -> (reference out=w268:refnum<vi>, error out=w269:errorcluster, "FP.State"=w267:T4)
            n78 = Not Equal?(x=w267, y=w265) -> (x != y?=w266:bool)
            n79 = case shown="True" w266 {
              tunnel: [w276 w278] -> w272
              tunnel: w269 -> [w275 w278]
              tunnel: w268 -> [w274 _]
              tunnel: w265 -> [w273 _]
              frame True {
                n80 = invoke class="VI" method="FP.Open"(reference=w274, error in=w275, "Activate"=TRUE, "State"=w273) -> (error out=w276:errorcluster)  [unwired: 1 in, 4 out]
              }
              frame False {
              }
            }
          }
          frame "Close", "Closed" {
            n81 = property class="VI"(reference=w283, error in=w285) -> (reference out=w282:refnum<vi>, error out=w284:errorcluster, "FP.State"=w280:T4)
            n82 = Not Equal?(x=w280, y=T4."Closed" ("Front Panel Window:State")) -> (x != y?=w279:bool)
            n83 = case shown="True" w279 {
              tunnel: [w287 w290] -> w286
              tunnel: w284 -> [w287 w289]
              tunnel: w282 -> [_ w288]
              frame False {
              }
              frame True {
                n84 = invoke class="VI" method="FP.Close"(reference=w288, error in=w289) -> (error out=w290:errorcluster)  [unwired: 1 in, 2 out]
              }
            }
          }
          frame "Hidden", "Hide" {
            w291 = T4."Hidden" ("State")
            n85 = property class="VI"(reference=w297, error in=w296) -> (reference out=w294:refnum<vi>, error out=w295:errorcluster, "FP.State"=w293:T4)
            n86 = Not Equal?(x=w293, y=w291) -> (x != y?=w292:bool)
            n87 = case shown="True" w292 {
              tunnel: [w302 w303] -> w298
              tunnel: w295 -> [w301 w303]
              tunnel: w294 -> [w300 _]
              tunnel: w291 -> [w299 _]
              frame True {
                n88 = invoke class="VI" method="FP.Open"(reference=w300, error in=w301, "State"=w299) -> (error out=w302:errorcluster)  [unwired: 2 in, 4 out]
              }
              frame False {
              }
            }
          }
          frame "Minimize", "Minimized" {
            w304 = T4."Minimized" ("State")
            n89 = property class="VI"(reference=w310, error in=w309) -> (reference out=w307:refnum<vi>, error out=w308:errorcluster, "FP.State"=w306:T4)
            n90 = Not Equal?(x=w306, y=w304) -> (x != y?=w305:bool)
            n91 = case shown="False" w305 {
              tunnel: [w315 w316] -> w311
              tunnel: w308 -> [w314 w316]
              tunnel: w307 -> [w313 _]
              tunnel: w304 -> [w312 _]
              frame True {
                n92 = invoke class="VI" method="FP.Open"(reference=w313, error in=w314, "State"=w312) -> (error out=w315:errorcluster)  [unwired: 2 in, 4 out]
              }
              frame False {
              }
            }
          }
          frame "Maximize", "Maximized" {
            w317 = T4."Maximized" ("State")
            n93 = property class="VI"(reference=w323, error in=w322) -> (reference out=w320:refnum<vi>, error out=w321:errorcluster, "FP.State"=w319:T4)
            n94 = Not Equal?(x=w319, y=w317) -> (x != y?=w318:bool)
            n95 = case shown="True" w318 {
              tunnel: [w328 w329] -> w324
              tunnel: w321 -> [w327 w329]
              tunnel: w320 -> [w326 _]
              tunnel: w317 -> [w325 _]
              frame True {
                n96 = invoke class="VI" method="FP.Open"(reference=w326, error in=w327, "State"=w325) -> (error out=w328:errorcluster)  [unwired: 2 in, 4 out]
              }
              frame False {
              }
            }
          }
        }
        n97 = call <vilib>:"Add State(s) to Queue__JKI_lib_State_Machine.vi"("State(s) in (\"\")"=w264) -> ("States Out"=w263:string)  [unwired: 14 in]
      }
      frame "---------- Macro ----------" {
        # "#CSM \"Category Seperator\"\nDo not put any code in this frame."
        n98 = call <vilib>:"Add State(s) to Queue__JKI_lib_State_Machine.vi"("State(s) in (\"\")"=w334) -> ("States Out"=w333:string)  [unwired: 14 in]
      }
      frame "Macro: Initialize" {
        w336 = "Data: Initialize\nInitialize Core Data\nEvents: Register\nUI: Initialize\nUI: Front Panel State >> Open"  # Data: Initialize Initialize Core Data Events: Register UI: Initialize UI: Front Panel State >> Open
        # "#CSM \"Macro: Initialize\"\nInitialization Macro (This is called once, when the VI starts)"
        n99 = call <vilib>:"Add State(s) to Queue__JKI_lib_State_Machine.vi"("State(s) in Front (\"\")"=w336, "State(s) in (\"\")"=w340) -> ("States Out"=w339:string)  [unwired: 13 in]
      }
      frame "Macro: Exit" {
        (unwired) "//Exit Other Modules \n//Macro: Exit -@ Chain\nMacro: Exit -@ Chain$1\nMacro: Exit -@ Chain$2\nMacro: Exit -@ Chain$3"
        # "#CSM \"Macro: Exit\"\nExit Macro (This is called once, when the VI exits)"
        n100 = Unbundle By Name(w350) -> ("Core.Close Panel on Exit?"=w349:bool)
        n101 = call "CSM - Build Exit Messages of CSMs.vi"("CSMs"=string[] ["Chain"]) -> ("States"=w341:string)  [unwired: 14 in]
        n102 = Select(t="UI: Front Panel State >> Close", s=w349, f="") -> (s? t:f=w346:string)
        n103 = call <vilib>:"Add State(s) to Queue__JKI_lib_State_Machine.vi"("State(s) in Front (\"\")"=w341, "State(s) in (\"\")"=w346, "State(s) at Back (\"\")"="Data: Cleanup\nEvents: Unregister\nExit") -> ("States Out"=w344:string)  [unwired: 12 in]
        n104 = call <vilib>:"Add State(s) to Queue__JKI_lib_State_Machine.vi"("State(s) in Front (\"\")"=w344, "State(s) in (\"\")"=w353) -> ("States Out"=w352:string)  [unwired: 13 in]
      }
      frame "---------- API ----------" {
        # "#CSM \"Category Seperator\"\nDo not put any code in this frame."
      }
      frame "API: API1" {
        # "#CSM >> From CSM >>\nIf you need to tell who triggered this state , use this string. If it's this case itself, this string is \"\"."
        # "#CSM >> Arguments >>\nDeal with the parameter if any"
        # "#CSM Response\nConnect this to return the response of your API"
        # "#CSM API Example\nCopy/Rename this case for your own API"
      }
      frame "API: API2" {
        # "#CSM API Example\nCopy/Rename this case for your own API"
      }
      frame "---------- DoSth ----------" {
        # "#CSM \"Category Seperator\"\nDo not put any code in this frame."
        n105 = call <vilib>:"Add State(s) to Queue__JKI_lib_State_Machine.vi"("State(s) in (\"\")"=w371) -> ("States Out"=w370:string)  [unwired: 14 in]
      }
      frame "DoSth: DoA" {
        # "#CSM \"Internal State\"\nThis category is used for holding internal states"
        n106 = call <vilib>:"Add State(s) to Queue__JKI_lib_State_Machine.vi"("State(s) in (\"\")"=w376) -> ("States Out"=w375:string)  [unwired: 14 in]
      }
      frame "DoSth: DoB" {
        # "#CSM \"Internal State\"\nThis category is used for holding internal states"
        n107 = call <vilib>:"Add State(s) to Queue__JKI_lib_State_Machine.vi"("State(s) in (\"\")"=w381) -> ("States Out"=w380:string)  [unwired: 14 in]
      }
    }
  }
  n108 = while {
    tunnel: w1 -> [w384]
    stop <- w385 stop-if-true
    n109 = call "CSM - Module Turns Invalid.vi"("CSM Name"=w384) -> ("Turn Invalid (Exit)?"=w385:bool)  [unwired: 2 in]
    n110 = call "CSM - List Modules.vi"("With Instance? (F)"="All?") -> ("Module Names"=w386:string[])  [unwired: 9 in, 1 out]
    n111 = for {
      tunnel: w386 -> [w394] mode=indexing
      tunnel: [w389] -> w387 mode=indexing
      n112 = call "CSM - Module Status.vi"("CSM Name"=w394) -> ("error out"=w388:errorcluster, "#Instance"=w391:i32, "Mode"=w392:T1, "CSM Name (Dup)"=w393:string, "#Elements In Queue"=w390:i32)  [unwired: 6 in]
      n113 = Bundle("CSM Name (Dup)"=w393, "Mode"=w392, "#Instance"=w391, "#Elements In Queue"=w390) -> (w389:T9)  [unwired: 1 in]
      n114 = call <vilib>:"Clear Errors.vi"("error in (no error)"=w388) -> ()  [unwired: 5 in, 2 out]
    }
    "Array" <- w387
    n115 = Wait (ms)(milliseconds to wait=u32 100) -> ()  [unwired: 1 out]
  }
  n116 = disable-structure shown="Default" {
    disable-tunnel: w1 -> [w395 _]
    frame condition #0 (active) {
      n117 = call "CSM - Global Log Queue.vi"() -> ("error out"=w398:errorcluster, "GlobalEvent Queue"=w396:refnum<queue>)  [unwired: 10 in]
      n118 = while {
        shift-right: [w424] -> w399
        shift-left: w398 -> [w421]
        shift-right: [w410] -> w397
        shift-left: w396 -> [w425]
        tunnel: w395 -> [w404]
        stop <- w400 stop-if-true
        # "#CSM\nCalc log handling speed"
        # "#CSM\nStop the loop if no alive modules"
        # "#CSM\nThis will help to reduce CPU Usage"
        n119 = Get Queue Status(queue=w425, error in (no error)=w421) -> (queue out=w423:refnum<queue>, error out=w422:errorcluster, # elements in queue=w406:i32)  [unwired: 1 in, 5 out]
        "LogInQ" <- w406
        n120 = call "Auto Processing Level.vi"("#Left In Q"=w406) -> ("LogInQ Changing Speed (#/s)"=→"LogInQ changing Speed(#/s)":dbl, "Level"=w405:T3)  [unwired: 8 in, 1 out]
        "Level" <- w405
        n121 = Dequeue Element(queue=w423, timeout in ms (-1)=100, error in (no error)=w422) -> (queue out=w410:refnum<queue>, element=w420:T11, timed out?=w412:bool, error out=w424:errorcluster)
        n122 = Not(x=w412) -> (.not. x?=w411:bool)
        n123 = call "Occurrence Speed Counter.vi"("Occured? (T)"=w411) -> ("Speed (#/s)"=→"log handling Speed(#/s)":dbl)  [unwired: 8 in, 2 out]
        n124 = feedback #1("" ("String Cache")) -> (w416:string)
        n125 = case shown="False" w412 {
          tunnel: w420 -> [w428 _]
          tunnel: [w427 w436] -> w417
          tunnel: w416 -> [_ w436]
          tunnel: w405 -> [w426 _]
          frame False {
            n126 = disable-structure shown="Enabled" {
              disable-tunnel: w428 -> [w431 w434]
              disable-tunnel: [w429 w435] -> w427
              disable-tunnel: w426 -> [_ w433]
              frame Disabled {
                # "#CSM \nno periodical filter"
                n127 = call "Global Log To String(Source Time).vi"("Log"=w431) -> ("Log String"=w430:string)  [unwired: 9 in]
                n128 = call "String History Cacher.vi"("String"=w430) -> ("String Cache"=w429:string)  [unwired: 10 in]
              }
              frame Enabled {
                n129 = call "Global Log History Cacher.vi"("Cross CSM Data"=w434, "Settings"=T10 {"threashold(#/s)"=0.5, "Check Peroid(s)"=5.0}, "Level (Normal)"=w433) -> ("String Cache"=w435:string)  [unwired: 12 in]
              }
            }
          }
          frame True {
          }
        }
        n130 = feedback-in #1(w417) -> ()
        n131 = call "CSM - List Modules.vi"() -> ("Module Names"=w415:string[])  [unwired: 10 in, 1 out]
        n132 = Empty Array?(array=w415) -> (empty?=w402:bool)
        n133 = call "Rising Edge.vi"("Signal"=w402) -> ("Rising Edge"=w401:bool)
        n134 = call "CSM - Module Turns Invalid.vi"("CSM Name"=w404) -> ("Turn Invalid (Exit)?"=w403:bool)  [unwired: 2 in]
        n135 = Compound Arithmetic op=OR(w424, w401, w403) -> (w408:bool)
        n136 = call "Exit With Empty Queue Check.vi"("Queue"=w410, "Stop"=w408) -> ("Exit"=w400:bool)  [unwired: 8 in, 1 out]
        n137 = call "Check Timeout.vi"() -> ("Timeout"=w418:bool)  [unwired: 8 in]
        n138 = Or(x=w400, y=w418) -> (x .or. y?=w409:bool)
        n139 = case shown="True" w409 {
          tunnel: w417 -> [_ w437]
          frame False {
          }
          frame True {
            "State History 2" <- w437
          }
        }
      }
      n140 = call "CSM - Destroy Global Log Queue.vi"("Error In"=w399, "Global Log Queue"=w397) -> ()  [unwired: 9 in, 1 out]
    }
    frame condition #1 {
    }
  }
  n141 = flat-sequence "Synchronized Call Modules" {
    frame #0 {
      n142 = call "ChainNode A.vi"("Name (\"\" to Use UUID)"="Chain$1" ("Name (\"\" to Use UUID)")) -> ()  [unwired: 11 in]
      n143 = call "ChainNode B.vi"("Name (\"\" to Use UUID)"="Chain$3" ("Name (\"\" to Use UUID)")) -> ()  [unwired: 11 in]
      n144 = call "ChainNode C.vi"("Name (\"\" to Use UUID)"="Chain$5" ("Name (\"\" to Use UUID)")) -> ()  [unwired: 11 in]
    }
  }
